vi "InitNoteHandling.vi"() -> ()   [LabVIEW 2023]
doc: "This VI initializes miscellaneous devices such as the compressor and any decorations."
uses:
  <vilib>/Rock Robotics/WPI/ThirdParty/REV Robotics/REVLib/Typedef/Spark MAX Idle Mode.ctl
  <vilib>/Rock Robotics/WPI/ThirdParty/REV Robotics/REVLib/Typedef/Spark MAX Limit Switch Polarity.ctl
  <vilib>/Rock Robotics/WPI/ThirdParty/REV Robotics/REVLib/Typedef/Spark MAX Limit Direction.ctl
  GlobalNoteHandling.vi
  <vilib>/Rock Robotics/SystemInterfaces/DIO/FPGA_DIOPWMChannel.ctl
panel:
  in  "Intake_Config":T1={"Future Proof Configs"=FALSE, "MotorOutputInverted"=1, "MotorOutputNeutralMode"=0, "MotorOutputDutyCycleNeutralDeadband"=0.0, "MotorOutputPeakForwardDutyCycle"=1.0, "MotorOutputPeakReverseDutyCycle"=-1.0, "CurrentLimitsStatorCurrentLimit"=0.0, "CurrentLimitsStatorCurrentLimitEnable"=FALSE, "CurrentLimitsSupplyCurrentLimit"=0.0, "CurrentLimitsSupplyCurrentLimitEnable"=FALSE, "CurrentLimitsSupplyCurrentThreshold"=0.0, "CurrentLimitsSupplyTimeThreshold"=0.0, "VoltageSupplyVoltageTimeConstant"=0.0, "VoltagePeakForwardVoltage"=16.0, "VoltagePeakReverseVoltage"=-16.0, "TorqueCurrentPeakForwardTorqueCurrent"=800.0, "TorqueCurrentPeakReverseTorqueCurrent"=-800.0, "TorqueCurrentTorqueNeutralDeadband"=0.0, "FeedbackFeedbackRotorOffset"=0.0, "FeedbackSensorToMechanismRatio"=1.0, "FeedbackRotorToSensorRatio"=1.0, "FeedbackFeedbackSensorSource"=0, "FeedbackFeedbackRemoteSensorID"=0, "DifferentialSensorsDifferentialSensorSource"=0, "DifferentialSensorsDifferentialTalonFXSensorID"=0, "DifferentialSensorsDifferentialRemoteSensorID"=0, "DifferentialConstantsPeakDifferentialDutyCycle"=2.0, "DifferentialConstantsPeakDifferentialVoltage"=32.0, "DifferentialConstantsPeakDifferentialTorqueCurrent"=1600.0, "OpenLoopRampsDutyCycleOpenLoopRampPeriod"=0.0, "OpenLoopRampsVoltageOpenLoopRampPeriod"=0.0, "OpenLoopRampsTorqueOpenLoopRampPeriod"=0.0, "ClosedLoopRampsDutyCycleClosedLoopRampPeriod"=0.0, "ClosedLoopRampsVoltageClosedLoopRampPeriod"=0.0, "ClosedLoopRampsTorqueClosedLoopRampPeriod"=0.0, "HardwareLimitSwitchForwardLimitType"=0, "HardwareLimitSwitchForwardLimitAutosetPositionEnable"=FALSE, "HardwareLimitSwitchForwardLimitAutosetPositionValue"=0.0, "HardwareLimitSwitchForwardLimitEnable"=TRUE, "HardwareLimitSwitchForwardLimitSource"=0, "HardwareLimitSwitchForwardLimitRemoteSensorID"=0, "HardwareLimitSwitchReverseLimitType"=0, "HardwareLimitSwitchReverseLimitAutosetPositionEnable"=FALSE, "HardwareLimitSwitchReverseLimitAutosetPositionValue"=0.0, "HardwareLimitSwitchReverseLimitEnable"=TRUE, "HardwareLimitSwitchReverseLimitSource"=0, "HardwareLimitSwitchReverseLimitRemoteSensorID"=0, "AudioBeepOnBoot"=TRUE, "AudioBeepOnConfig"=TRUE, "AudioAllowMusicDurDisable"=FALSE, "SoftwareLimitSwitchForwardSoftLimitEnable"=FALSE, "SoftwareLimitSwitchReverseSoftLimitEnable"=FALSE, "SoftwareLimitSwitchForwardSoftLimitThreshold"=0.0, "SoftwareLimitSwitchReverseSoftLimitThreshold"=0.0, "MotionMagicMotionMagicCruiseVelocity"=0.0, "MotionMagicMotionMagicAcceleration"=0.0, "MotionMagicMotionMagicJerk"=0.0, "MotionMagicMotionMagicExpo_kV"=0.0, "MotionMagicMotionMagicExpo_kA"=0.0, "CustomParamsCustomParam0"=0, "CustomParamsCustomParam1"=0, "ClosedLoopGeneralContinuousWrap"=FALSE, "Slot0kP"=0.0, "Slot0kI"=0.0, "Slot0kD"=0.0, "Slot0kS"=0.0, "Slot0kV"=0.0, "Slot0kA"=0.0, "Slot0kG"=0.0, "Slot0GravityType"=0, "Slot0StaticFeedforwardSign"=0, "Slot1kP"=0.0, "Slot1kI"=0.0, "Slot1kD"=0.0, "Slot1kS"=0.0, "Slot1kV"=0.0, "Slot1kA"=0.0, "Slot1kG"=0.0, "Slot1GravityType"=0, "Slot1StaticFeedforwardSign"=0, "Slot2kP"=0.0, "Slot2kI"=0.0, "Slot2kD"=0.0, "Slot2kS"=0.0, "Slot2kV"=0.0, "Slot2kA"=0.0, "Slot2kG"=0.0, "Slot2GravityType"=0, "Slot2StaticFeedforwardSign"=0} {"MotorOutputInverted" items=["CounterClockwise_Positive", "Clockwise_Positive"]; "MotorOutputNeutralMode" items=["Coast", "Brake"]; "FeedbackFeedbackSensorSource" items=["RotorSensor", "RemoteCANcoder", "RemotePigeon2_Yaw", "RemotePigeon2_Pitch", "RemotePigeon2_Roll", "FusedCANcoder", "SyncCANcoder"]; "DifferentialSensorsDifferentialSensorSource" items=["Disabled", "RemoteTalonFX_Diff", "RemotePigeon2_Yaw", "RemotePigeon2_Pitch", "RemotePigeon2_Roll", "RemoteCANcoder"]; "HardwareLimitSwitchForwardLimitType" items=["NormallyOpen", "NormallyClosed"]; "HardwareLimitSwitchForwardLimitSource" items=["LimitSwitchPin"=0, "RemoteTalonFX"=1, "RemoteCANifier"=2, "RemoteCANcoder"=4, "Disabled"=3]; "HardwareLimitSwitchReverseLimitType" items=["NormallyOpen", "NormallyClosed"]; "HardwareLimitSwitchReverseLimitSource" items=["LimitSwitchPin"=0, "RemoteTalonFX"=1, "RemoteCANifier"=2, "RemoteCANcoder"=4, "Disabled"=3]; "Slot0GravityType" items=["Elevator_Static", "Arm_Cosine"]; "Slot0StaticFeedforwardSign" items=["UseVelocitySign", "UseClosedLoopSign"]; "Slot1GravityType" items=["Elevator_Static", "Arm_Cosine"]; "Slot1StaticFeedforwardSign" items=["UseVelocitySign", "UseClosedLoopSign"]; "Slot2GravityType" items=["Elevator_Static", "Arm_Cosine"]; "Slot2StaticFeedforwardSign" items=["UseVelocitySign", "UseClosedLoopSign"]}
  in  "Outer_Roller_Back_Config":T1={"Future Proof Configs"=FALSE, "MotorOutputInverted"=0, "MotorOutputNeutralMode"=0, "MotorOutputDutyCycleNeutralDeadband"=0.0, "MotorOutputPeakForwardDutyCycle"=1.0, "MotorOutputPeakReverseDutyCycle"=-1.0, "CurrentLimitsStatorCurrentLimit"=0.0, "CurrentLimitsStatorCurrentLimitEnable"=FALSE, "CurrentLimitsSupplyCurrentLimit"=0.0, "CurrentLimitsSupplyCurrentLimitEnable"=FALSE, "CurrentLimitsSupplyCurrentThreshold"=0.0, "CurrentLimitsSupplyTimeThreshold"=0.0, "VoltageSupplyVoltageTimeConstant"=0.0, "VoltagePeakForwardVoltage"=16.0, "VoltagePeakReverseVoltage"=-16.0, "TorqueCurrentPeakForwardTorqueCurrent"=800.0, "TorqueCurrentPeakReverseTorqueCurrent"=-800.0, "TorqueCurrentTorqueNeutralDeadband"=0.0, "FeedbackFeedbackRotorOffset"=0.0, "FeedbackSensorToMechanismRatio"=1.0, "FeedbackRotorToSensorRatio"=1.0, "FeedbackFeedbackSensorSource"=0, "FeedbackFeedbackRemoteSensorID"=0, "DifferentialSensorsDifferentialSensorSource"=0, "DifferentialSensorsDifferentialTalonFXSensorID"=0, "DifferentialSensorsDifferentialRemoteSensorID"=0, "DifferentialConstantsPeakDifferentialDutyCycle"=2.0, "DifferentialConstantsPeakDifferentialVoltage"=32.0, "DifferentialConstantsPeakDifferentialTorqueCurrent"=1600.0, "OpenLoopRampsDutyCycleOpenLoopRampPeriod"=0.0, "OpenLoopRampsVoltageOpenLoopRampPeriod"=0.0, "OpenLoopRampsTorqueOpenLoopRampPeriod"=0.0, "ClosedLoopRampsDutyCycleClosedLoopRampPeriod"=0.0, "ClosedLoopRampsVoltageClosedLoopRampPeriod"=0.0, "ClosedLoopRampsTorqueClosedLoopRampPeriod"=0.0, "HardwareLimitSwitchForwardLimitType"=0, "HardwareLimitSwitchForwardLimitAutosetPositionEnable"=FALSE, "HardwareLimitSwitchForwardLimitAutosetPositionValue"=0.0, "HardwareLimitSwitchForwardLimitEnable"=TRUE, "HardwareLimitSwitchForwardLimitSource"=0, "HardwareLimitSwitchForwardLimitRemoteSensorID"=0, "HardwareLimitSwitchReverseLimitType"=0, "HardwareLimitSwitchReverseLimitAutosetPositionEnable"=FALSE, "HardwareLimitSwitchReverseLimitAutosetPositionValue"=0.0, "HardwareLimitSwitchReverseLimitEnable"=TRUE, "HardwareLimitSwitchReverseLimitSource"=0, "HardwareLimitSwitchReverseLimitRemoteSensorID"=0, "AudioBeepOnBoot"=TRUE, "AudioBeepOnConfig"=TRUE, "AudioAllowMusicDurDisable"=FALSE, "SoftwareLimitSwitchForwardSoftLimitEnable"=FALSE, "SoftwareLimitSwitchReverseSoftLimitEnable"=FALSE, "SoftwareLimitSwitchForwardSoftLimitThreshold"=0.0, "SoftwareLimitSwitchReverseSoftLimitThreshold"=0.0, "MotionMagicMotionMagicCruiseVelocity"=0.0, "MotionMagicMotionMagicAcceleration"=0.0, "MotionMagicMotionMagicJerk"=0.0, "MotionMagicMotionMagicExpo_kV"=0.0, "MotionMagicMotionMagicExpo_kA"=0.0, "CustomParamsCustomParam0"=0, "CustomParamsCustomParam1"=0, "ClosedLoopGeneralContinuousWrap"=FALSE, "Slot0kP"=0.0, "Slot0kI"=0.0, "Slot0kD"=0.0, "Slot0kS"=0.0, "Slot0kV"=0.0, "Slot0kA"=0.0, "Slot0kG"=0.0, "Slot0GravityType"=0, "Slot0StaticFeedforwardSign"=0, "Slot1kP"=0.0, "Slot1kI"=0.0, "Slot1kD"=0.0, "Slot1kS"=0.0, "Slot1kV"=0.0, "Slot1kA"=0.0, "Slot1kG"=0.0, "Slot1GravityType"=0, "Slot1StaticFeedforwardSign"=0, "Slot2kP"=0.0, "Slot2kI"=0.0, "Slot2kD"=0.0, "Slot2kS"=0.0, "Slot2kV"=0.0, "Slot2kA"=0.0, "Slot2kG"=0.0, "Slot2GravityType"=0, "Slot2StaticFeedforwardSign"=0} {"MotorOutputInverted" items=["CounterClockwise_Positive", "Clockwise_Positive"]; "MotorOutputNeutralMode" items=["Coast", "Brake"]; "FeedbackFeedbackSensorSource" items=["RotorSensor", "RemoteCANcoder", "RemotePigeon2_Yaw", "RemotePigeon2_Pitch", "RemotePigeon2_Roll", "FusedCANcoder", "SyncCANcoder"]; "DifferentialSensorsDifferentialSensorSource" items=["Disabled", "RemoteTalonFX_Diff", "RemotePigeon2_Yaw", "RemotePigeon2_Pitch", "RemotePigeon2_Roll", "RemoteCANcoder"]; "HardwareLimitSwitchForwardLimitType" items=["NormallyOpen", "NormallyClosed"]; "HardwareLimitSwitchForwardLimitSource" items=["LimitSwitchPin"=0, "RemoteTalonFX"=1, "RemoteCANifier"=2, "RemoteCANcoder"=4, "Disabled"=3]; "HardwareLimitSwitchReverseLimitType" items=["NormallyOpen", "NormallyClosed"]; "HardwareLimitSwitchReverseLimitSource" items=["LimitSwitchPin"=0, "RemoteTalonFX"=1, "RemoteCANifier"=2, "RemoteCANcoder"=4, "Disabled"=3]; "Slot0GravityType" items=["Elevator_Static", "Arm_Cosine"]; "Slot0StaticFeedforwardSign" items=["UseVelocitySign", "UseClosedLoopSign"]; "Slot1GravityType" items=["Elevator_Static", "Arm_Cosine"]; "Slot1StaticFeedforwardSign" items=["UseVelocitySign", "UseClosedLoopSign"]; "Slot2GravityType" items=["Elevator_Static", "Arm_Cosine"]; "Slot2StaticFeedforwardSign" items=["UseVelocitySign", "UseClosedLoopSign"]}
  in  "Outer_Roller_Front_Config":T1={"Future Proof Configs"=FALSE, "MotorOutputInverted"=0, "MotorOutputNeutralMode"=0, "MotorOutputDutyCycleNeutralDeadband"=0.0, "MotorOutputPeakForwardDutyCycle"=1.0, "MotorOutputPeakReverseDutyCycle"=-1.0, "CurrentLimitsStatorCurrentLimit"=0.0, "CurrentLimitsStatorCurrentLimitEnable"=FALSE, "CurrentLimitsSupplyCurrentLimit"=0.0, "CurrentLimitsSupplyCurrentLimitEnable"=FALSE, "CurrentLimitsSupplyCurrentThreshold"=0.0, "CurrentLimitsSupplyTimeThreshold"=0.0, "VoltageSupplyVoltageTimeConstant"=0.0, "VoltagePeakForwardVoltage"=16.0, "VoltagePeakReverseVoltage"=-16.0, "TorqueCurrentPeakForwardTorqueCurrent"=800.0, "TorqueCurrentPeakReverseTorqueCurrent"=-800.0, "TorqueCurrentTorqueNeutralDeadband"=0.0, "FeedbackFeedbackRotorOffset"=0.0, "FeedbackSensorToMechanismRatio"=1.0, "FeedbackRotorToSensorRatio"=1.0, "FeedbackFeedbackSensorSource"=0, "FeedbackFeedbackRemoteSensorID"=0, "DifferentialSensorsDifferentialSensorSource"=0, "DifferentialSensorsDifferentialTalonFXSensorID"=0, "DifferentialSensorsDifferentialRemoteSensorID"=0, "DifferentialConstantsPeakDifferentialDutyCycle"=2.0, "DifferentialConstantsPeakDifferentialVoltage"=32.0, "DifferentialConstantsPeakDifferentialTorqueCurrent"=1600.0, "OpenLoopRampsDutyCycleOpenLoopRampPeriod"=0.0, "OpenLoopRampsVoltageOpenLoopRampPeriod"=0.0, "OpenLoopRampsTorqueOpenLoopRampPeriod"=0.0, "ClosedLoopRampsDutyCycleClosedLoopRampPeriod"=0.0, "ClosedLoopRampsVoltageClosedLoopRampPeriod"=0.0, "ClosedLoopRampsTorqueClosedLoopRampPeriod"=0.0, "HardwareLimitSwitchForwardLimitType"=0, "HardwareLimitSwitchForwardLimitAutosetPositionEnable"=FALSE, "HardwareLimitSwitchForwardLimitAutosetPositionValue"=0.0, "HardwareLimitSwitchForwardLimitEnable"=TRUE, "HardwareLimitSwitchForwardLimitSource"=0, "HardwareLimitSwitchForwardLimitRemoteSensorID"=0, "HardwareLimitSwitchReverseLimitType"=0, "HardwareLimitSwitchReverseLimitAutosetPositionEnable"=FALSE, "HardwareLimitSwitchReverseLimitAutosetPositionValue"=0.0, "HardwareLimitSwitchReverseLimitEnable"=TRUE, "HardwareLimitSwitchReverseLimitSource"=0, "HardwareLimitSwitchReverseLimitRemoteSensorID"=0, "AudioBeepOnBoot"=TRUE, "AudioBeepOnConfig"=TRUE, "AudioAllowMusicDurDisable"=FALSE, "SoftwareLimitSwitchForwardSoftLimitEnable"=FALSE, "SoftwareLimitSwitchReverseSoftLimitEnable"=FALSE, "SoftwareLimitSwitchForwardSoftLimitThreshold"=0.0, "SoftwareLimitSwitchReverseSoftLimitThreshold"=0.0, "MotionMagicMotionMagicCruiseVelocity"=0.0, "MotionMagicMotionMagicAcceleration"=0.0, "MotionMagicMotionMagicJerk"=0.0, "MotionMagicMotionMagicExpo_kV"=0.0, "MotionMagicMotionMagicExpo_kA"=0.0, "CustomParamsCustomParam0"=0, "CustomParamsCustomParam1"=0, "ClosedLoopGeneralContinuousWrap"=FALSE, "Slot0kP"=0.0, "Slot0kI"=0.0, "Slot0kD"=0.0, "Slot0kS"=0.0, "Slot0kV"=0.0, "Slot0kA"=0.0, "Slot0kG"=0.0, "Slot0GravityType"=0, "Slot0StaticFeedforwardSign"=0, "Slot1kP"=0.0, "Slot1kI"=0.0, "Slot1kD"=0.0, "Slot1kS"=0.0, "Slot1kV"=0.0, "Slot1kA"=0.0, "Slot1kG"=0.0, "Slot1GravityType"=0, "Slot1StaticFeedforwardSign"=0, "Slot2kP"=0.0, "Slot2kI"=0.0, "Slot2kD"=0.0, "Slot2kS"=0.0, "Slot2kV"=0.0, "Slot2kA"=0.0, "Slot2kG"=0.0, "Slot2GravityType"=0, "Slot2StaticFeedforwardSign"=0} {"MotorOutputInverted" items=["CounterClockwise_Positive", "Clockwise_Positive"]; "MotorOutputNeutralMode" items=["Coast", "Brake"]; "FeedbackFeedbackSensorSource" items=["RotorSensor", "RemoteCANcoder", "RemotePigeon2_Yaw", "RemotePigeon2_Pitch", "RemotePigeon2_Roll", "FusedCANcoder", "SyncCANcoder"]; "DifferentialSensorsDifferentialSensorSource" items=["Disabled", "RemoteTalonFX_Diff", "RemotePigeon2_Yaw", "RemotePigeon2_Pitch", "RemotePigeon2_Roll", "RemoteCANcoder"]; "HardwareLimitSwitchForwardLimitType" items=["NormallyOpen", "NormallyClosed"]; "HardwareLimitSwitchForwardLimitSource" items=["LimitSwitchPin"=0, "RemoteTalonFX"=1, "RemoteCANifier"=2, "RemoteCANcoder"=4, "Disabled"=3]; "HardwareLimitSwitchReverseLimitType" items=["NormallyOpen", "NormallyClosed"]; "HardwareLimitSwitchReverseLimitSource" items=["LimitSwitchPin"=0, "RemoteTalonFX"=1, "RemoteCANifier"=2, "RemoteCANcoder"=4, "Disabled"=3]; "Slot0GravityType" items=["Elevator_Static", "Arm_Cosine"]; "Slot0StaticFeedforwardSign" items=["UseVelocitySign", "UseClosedLoopSign"]; "Slot1GravityType" items=["Elevator_Static", "Arm_Cosine"]; "Slot1StaticFeedforwardSign" items=["UseVelocitySign", "UseClosedLoopSign"]; "Slot2GravityType" items=["Elevator_Static", "Arm_Cosine"]; "Slot2StaticFeedforwardSign" items=["UseVelocitySign", "UseClosedLoopSign"]}
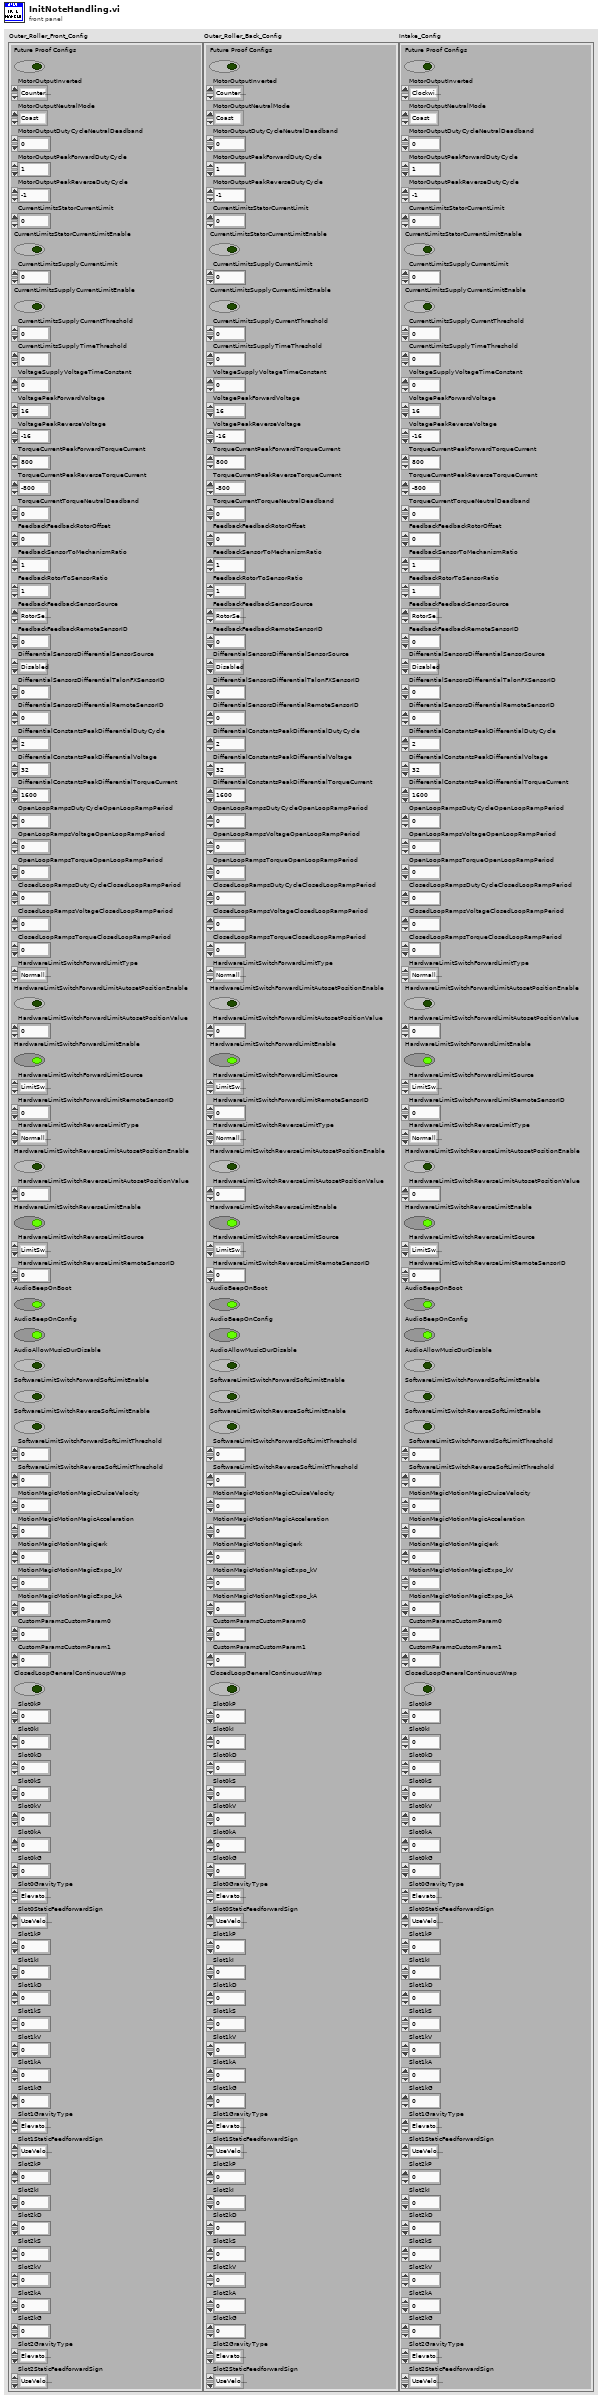
[diagram p1: front panel]
types:
  T1 = cluster{"Future Proof Configs":bool, "MotorOutputInverted":u16, "MotorOutputNeutralMode":u16, "MotorOutputDutyCycleNeutralDeadband":dbl, "MotorOutputPeakForwardDutyCycle":dbl, "MotorOutputPeakReverseDutyCycle":dbl, "CurrentLimitsStatorCurrentLimit":dbl, "CurrentLimitsStatorCurrentLimitEnable":bool, "CurrentLimitsSupplyCurrentLimit":dbl, "CurrentLimitsSupplyCurrentLimitEnable":bool, "CurrentLimitsSupplyCurrentThreshold":dbl, "CurrentLimitsSupplyTimeThreshold":dbl, "VoltageSupplyVoltageTimeConstant":dbl, "VoltagePeakForwardVoltage":dbl, "VoltagePeakReverseVoltage":dbl, "TorqueCurrentPeakForwardTorqueCurrent":dbl, "TorqueCurrentPeakReverseTorqueCurrent":dbl, "TorqueCurrentTorqueNeutralDeadband":dbl, "FeedbackFeedbackRotorOffset":dbl, "FeedbackSensorToMechanismRatio":dbl, "FeedbackRotorToSensorRatio":dbl, "FeedbackFeedbackSensorSource":u16, "FeedbackFeedbackRemoteSensorID":i16, "DifferentialSensorsDifferentialSensorSource":u16, "DifferentialSensorsDifferentialTalonFXSensorID":i16, "DifferentialSensorsDifferentialRemoteSensorID":i16, "DifferentialConstantsPeakDifferentialDutyCycle":dbl, "DifferentialConstantsPeakDifferentialVoltage":dbl, "DifferentialConstantsPeakDifferentialTorqueCurrent":dbl, "OpenLoopRampsDutyCycleOpenLoopRampPeriod":dbl, "OpenLoopRampsVoltageOpenLoopRampPeriod":dbl, "OpenLoopRampsTorqueOpenLoopRampPeriod":dbl, "ClosedLoopRampsDutyCycleClosedLoopRampPeriod":dbl, "ClosedLoopRampsVoltageClosedLoopRampPeriod":dbl, "ClosedLoopRampsTorqueClosedLoopRampPeriod":dbl, "HardwareLimitSwitchForwardLimitType":u16, "HardwareLimitSwitchForwardLimitAutosetPositionEnable":bool, "HardwareLimitSwitchForwardLimitAutosetPositionValue":dbl, "HardwareLimitSwitchForwardLimitEnable":bool, "HardwareLimitSwitchForwardLimitSource":u16, "HardwareLimitSwitchForwardLimitRemoteSensorID":i16, "HardwareLimitSwitchReverseLimitType":u16, "HardwareLimitSwitchReverseLimitAutosetPositionEnable":bool, "HardwareLimitSwitchReverseLimitAutosetPositionValue":dbl, "HardwareLimitSwitchReverseLimitEnable":bool, "HardwareLimitSwitchReverseLimitSource":u16, "HardwareLimitSwitchReverseLimitRemoteSensorID":i16, "AudioBeepOnBoot":bool, "AudioBeepOnConfig":bool, "AudioAllowMusicDurDisable":bool, "SoftwareLimitSwitchForwardSoftLimitEnable":bool, "SoftwareLimitSwitchReverseSoftLimitEnable":bool, "SoftwareLimitSwitchForwardSoftLimitThreshold":dbl, "SoftwareLimitSwitchReverseSoftLimitThreshold":dbl, "MotionMagicMotionMagicCruiseVelocity":dbl, "MotionMagicMotionMagicAcceleration":dbl, "MotionMagicMotionMagicJerk":dbl, "MotionMagicMotionMagicExpo_kV":dbl, "MotionMagicMotionMagicExpo_kA":dbl, "CustomParamsCustomParam0":i16, "CustomParamsCustomParam1":i16, "ClosedLoopGeneralContinuousWrap":bool, "Slot0kP":dbl, "Slot0kI":dbl, "Slot0kD":dbl, "Slot0kS":dbl, "Slot0kV":dbl, "Slot0kA":dbl, "Slot0kG":dbl, "Slot0GravityType":u16, "Slot0StaticFeedforwardSign":u16, "Slot1kP":dbl, "Slot1kI":dbl, "Slot1kD":dbl, "Slot1kS":dbl, "Slot1kV":dbl, "Slot1kA":dbl, "Slot1kG":dbl, "Slot1GravityType":u16, "Slot1StaticFeedforwardSign":u16, "Slot2kP":dbl, "Slot2kI":dbl, "Slot2kD":dbl, "Slot2kS":dbl, "Slot2kV":dbl, "Slot2kA":dbl, "Slot2kG":dbl, "Slot2GravityType":u16, "Slot2StaticFeedforwardSign":u16}
  T2 = typedef "Spark MAX Limit Direction.ctl" = enum16{"Forward Limit", "Reverse Limit"}
  T3 = typedef "Spark MAX Limit Switch Polarity.ctl" = enum16{"Normally Open", "Normally Closed"}
  T4 = typedef "Spark MAX Idle Mode.ctl" = enum16{"Coast", "Brake"}
  T5 = typedef "WPI_MotorControlDeviceRef.ctl" = cluster{"DeviceStatus":errorcluster, "Type":T6, "PWM":cluster{"PWM Channel":T7, "DeadBand":T8}, "CAN":cluster{"Device Number":u8, "SetOutput VI Ref":variant, "GetOutput VI Ref":variant, "Enable VI Ref":variant, "Disable VI Ref":variant, "Data":variant}, "Invert":bool, "DIO PWM":cluster{"PWM \"Enable\" Channel":T7, "DIOChannel":T9, "PWM Rate":dbl}}
  T6 = typedef "WPI_MotorControlType.ctl" = enum16{"PWM", "CAN", "DIO PWM"}
  T7 = typedef "FPGA_DIOPWMChannel.ctl" = enum8{"PWM 0", "PWM 1", "PWM 2", "PWM 3", "PWM 4", "PWM 5", "PWM 6", "PWM 7", "PWM 8", "PWM 9", "PWM MXP 0", "PWM MXP 1", "PWM MXP 2", "PWM MXP 3", "PWM MXP 4", "PWM MXP 5", "PWM MXP 6", "PWM MXP 7", "PWM MXP 8", "PWM MXP 9", "Invalid"}
  T8 = typedef "WPI_PWMDeadband.ctl" = cluster{"Name":string, "maxPositivePwm":i32, "minPositivePwm":i32, "centerPwm":i32, "maxNegativePwm":i32, "minNegativePwm":i32, "angularRange":u16}
  T9 = typedef "FPGA_DIOChannel.ctl" = enum8{"DIO 0", "DIO 1", "DIO 2", "DIO 3", "DIO 4", "DIO 5", "DIO 6", "DIO 7", "DIO 8", "DIO 9", "DIO MXP 0", "DIO MXP 1", "DIO MXP 2", "DIO MXP 3", "DIO MXP 4", "DIO MXP 5", "DIO MXP 6", "DIO MXP 7", "DIO MXP 8", "DIO MXP 9", "DIO MXP 10", "DIO MXP 11", "DIO MXP 12", "DIO MXP 13", "DIO MXP 14", "DIO MXP 15", "SPI Port CS1", "SPI Port CS2", "SPI Port CS3", "SPI Port MISO", "SPI Port MOSI", "Invalid"}
  T10 = typedef "DeviceReference.ctl" = cluster{"CANbus Name":string, "Device Encoding":u32, "Device Name":string}
  T11 = typedef "WPI_ServoDeviceRef.ctl" = cluster{"DeviceStatus":errorcluster, "PWM Channel":T7, "DeadBand":T8}
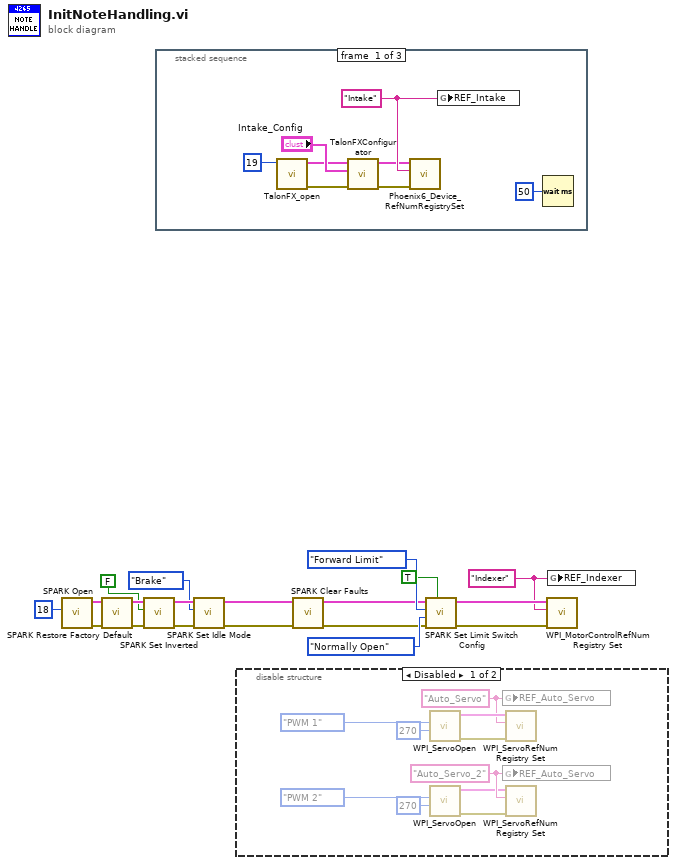
[diagram p0: block diagram]
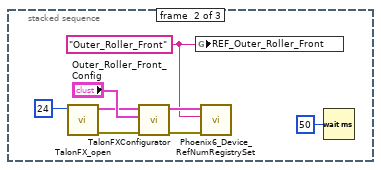
[diagram p2: hidden frame]
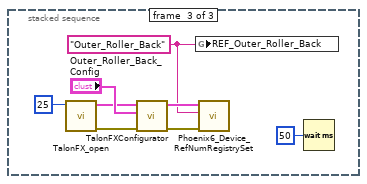
[diagram p3: hidden frame]
diagram:
  w6 = "Indexer" ("refnum name")
  n1 = call <vilib>:"SPARK Open.vi"("Device Number"=u8 18) -> ("error out"=w17:errorcluster, "MotorControlDeviceRef"=w18:T5)  [unwired: 9 in]
  n2 = call <vilib>:"SPARK Restore Factory Default.vi"("error in"=w17, "MotorControlDeviceRef"=w18) -> ("error out"=w16:errorcluster, "MotorControlDeviceRef"=w15:T5)  [unwired: 8 in]
  n3 = call <vilib>:"SPARK Set Inverted.vi"("error in (no error)"=w16, "Inverted (F)"=FALSE, "MotorControlDeviceRef in"=w15) -> ("error out"=w12:errorcluster, "MotorControlDeviceRef out"=w13:T5)  [unwired: 7 in]
  n4 = stacked-sequence {
    frame #0 {
      w25 = "Intake" ("refnum name")
      n5 = call <vilib>:"TalonFX_open.vi"("Device ID"=u8 19 ("Device Number")) -> ("error out"=w24:errorcluster, "DeviceReference 2"=w22:T10)  [unwired: 9 in]
      n6 = call <vilib>:"TalonFXConfigurator.vi"("error in"=w24, "DeviceConfiguration"="Intake_Config", "DeviceReference"=w22) -> ("error out"=w21:errorcluster)  [unwired: 8 in]
      n7 = call <vilib>:"Phoenix6_Device_RefNumRegistrySet.vi"("error in (no error)"=w21, "refnum name"=w25, "DeviceReference"=w22) -> ()  [unwired: 7 in, 2 out]
      n8 = global write "GlobalNoteHandling.vi" "REF_Intake"(w25) -> ()
      n9 = Wait (ms)(milliseconds to wait=u32 50) -> ()  [unwired: 1 out]
    }
    frame #1 {
      w29 = "Outer_Roller_Front" ("refnum name")
      n10 = call <vilib>:"TalonFX_open.vi"("Device ID"=u8 24 ("Device Number")) -> ("error out"=w33:errorcluster, "DeviceReference 2"=w31:T10)  [unwired: 9 in]
      n11 = call <vilib>:"TalonFXConfigurator.vi"("error in"=w33, "DeviceConfiguration"="Outer_Roller_Front_Config", "DeviceReference"=w31) -> ("error out"=w30:errorcluster)  [unwired: 8 in]
      n12 = global write "GlobalNoteHandling.vi" "REF_Outer_Roller_Front"(w29) -> ()
      n13 = call <vilib>:"Phoenix6_Device_RefNumRegistrySet.vi"("error in (no error)"=w30, "refnum name"=w29, "DeviceReference"=w31) -> ()  [unwired: 7 in, 2 out]
      n14 = Wait (ms)(milliseconds to wait=u32 50) -> ()  [unwired: 1 out]
    }
    frame #2 {
      w36 = "Outer_Roller_Back" ("refnum name")
      n15 = call <vilib>:"TalonFX_open.vi"("Device ID"=u8 25 ("Device Number")) -> ("error out"=w40:errorcluster, "DeviceReference 2"=w38:T10)  [unwired: 9 in]
      n16 = call <vilib>:"TalonFXConfigurator.vi"("error in"=w40, "DeviceConfiguration"="Outer_Roller_Back_Config", "DeviceReference"=w38) -> ("error out"=w37:errorcluster)  [unwired: 8 in]
      n17 = global write "GlobalNoteHandling.vi" "REF_Outer_Roller_Back"(w36) -> ()
      n18 = call <vilib>:"Phoenix6_Device_RefNumRegistrySet.vi"("error in (no error)"=w37, "refnum name"=w36, "DeviceReference"=w38) -> ()  [unwired: 7 in, 2 out]
      n19 = Wait (ms)(milliseconds to wait=u32 50) -> ()  [unwired: 1 out]
    }
  }
  n20 = call <vilib>:"SPARK Set Idle Mode.vi"("error in (no error)"=w12, "Idle Mode"=Spark_MAX_Idle_Mode."Brake", "MotorControlDeviceRef in"=w13) -> ("error out"=w4:errorcluster, "MotorControlDeviceRef out"=w5:T5)  [unwired: 7 in]
  n21 = disable-structure shown="Disabled" {
    frame Disabled {
      w45 = "Auto_Servo_2" ("refnum name")
      w46 = "Auto_Servo" ("refnum name")
      n22 = call <vilib>:"WPI_ServoOpen.vi"("Angular Range"=u16 270, "PWM Channel"=FPGA_DIOPWMChannel."PWM 1") -> ("error out"=w47:errorcluster, "ServoDeviceRef"=w48:T11)  [unwired: 8 in]
      n23 = call <vilib>:"WPI_ServoOpen.vi"("Angular Range"=u16 270, "PWM Channel"=FPGA_DIOPWMChannel."PWM 2") -> ("error out"=w44:errorcluster, "ServoDeviceRef"=w43:T11)  [unwired: 8 in]
      n24 = global write "GlobalNoteHandling.vi" "REF_Auto_Servo"(w46) -> ()
      n25 = global write "GlobalNoteHandling.vi" "REF_Auto_Servo"(w45) -> ()
      n26 = call <vilib>:"WPI_ServoRefNum Registry Set.vi"("error in (no error)"=w47, "refnum name"=w46, "ServoDeviceRef"=w48) -> ()  [unwired: 7 in, 2 out]
      n27 = call <vilib>:"WPI_ServoRefNum Registry Set.vi"("error in (no error)"=w44, "refnum name"=w45, "ServoDeviceRef"=w43) -> ()  [unwired: 7 in, 2 out]
    }
    frame Enabled {
    }
  }
  n28 = call <vilib>:"SPARK Clear Faults.vi"("error in"=w4, "MotorControlDeviceRef"=w5) -> ("error out"=w3:errorcluster, "MotorControlDeviceRef"=w2:T5)  [unwired: 8 in]
  n29 = call <vilib>:"SPARK Set Limit Switch Config.vi"("Enabled? (T)"=TRUE, "error in (no error)"=w3, "Polarity (Normally Open)"=Spark_MAX_Limit_Switch_Polarity."Normally Open", "Limit Switch"=Spark_MAX_Limit_Direction."Forward Limit", "MotorControlDeviceRef in"=w2) -> ("error out"=w8:errorcluster, "MotorControlDeviceRef out"=w7:T5)  [unwired: 5 in]
  n30 = call <vilib>:"WPI_MotorControlRefNum Registry Set.vi"("error in (no error)"=w8, "refnum name"=w6, "MotorControlDevRef"=w7) -> ()  [unwired: 7 in, 2 out]
  n31 = global write "GlobalNoteHandling.vi" "REF_Indexer"(w6) -> ()
